vi "Thin Etalon Linewidth Sweep 2.0 user.vi"() -> ()   [LabVIEW 2013]
uses:
  Sweep Control.ctl
panel:
  out "time":dbl(graph)
  out "centers":T1(graph)
  out "Remote Find Center":bool
  out "sweep states":T2
  out "Loop Counter":i32
  in  "Stop Button":bool
  out "Done":bool
  in  "Find Center":bool
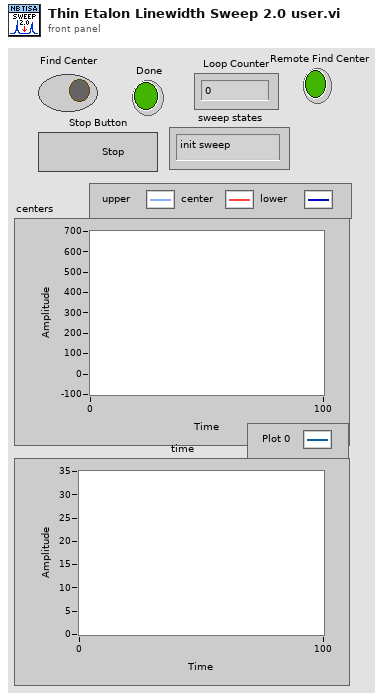
[diagram p1: front panel]
types:
  T1 = cluster{"Upper Limit":i32, "Center Position":i32, "Lower Limit":i32}
  T2 = typedef "Sweep Control.ctl" = enum16{"init sweep", "do sweep", "idle"}
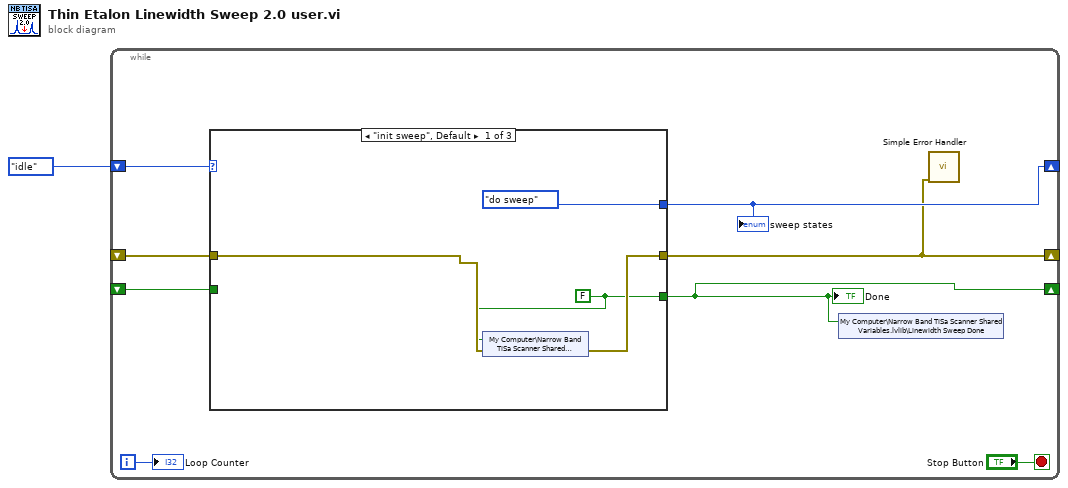
[diagram p0: block diagram]
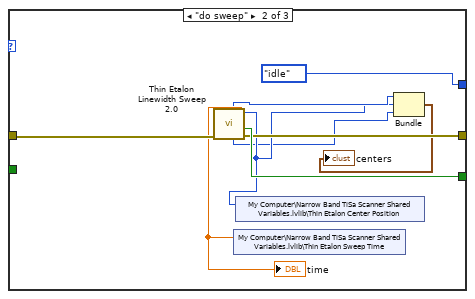
[diagram p2: hidden frame]
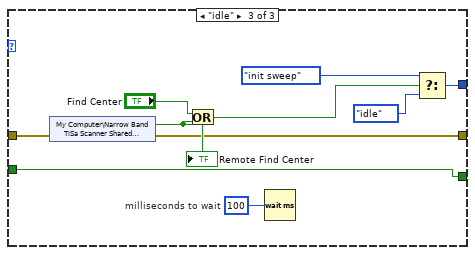
[diagram p3: hidden frame]
diagram:
  n1 = while {
    shift-right: [w5] -> _
    shift-left: Sweep_Control."idle" -> [w7]
    shift-right: [w2] -> _
    shift-left: _ -> [w6]
    shift-right: [w4] -> _
    shift-left: _ -> [w3]
    i -> [w8]
    stop <- "Stop Button" stop-if-true
    n2 = case shown="\"init sweep\", Default" w7 {
      tunnel: [w11 w20 w23] -> w2
      tunnel: w6 -> [w12 w21 w30]
      tunnel: [Sweep_Control."do sweep" Sweep_Control."idle" w26] -> w5
      tunnel: [w10 w22 w24] -> w4
      tunnel: w3 -> [_ _ w24]
      frame "init sweep", Default {
        w10 = FALSE
        n3 = shared-variable "My Computer\\Narrow Band TiSa Scanner Shared Variables.lvlib\\Find Center"(w10, error in=w12) -> (error out=w11:errorcluster)
      }
      frame "do sweep" {
        n4 = call "Thin Etalon Linewidth Sweep 2.0.vi"("Error In"=w21) -> ("Error Out"=w20:errorcluster, "Done"=w22:bool, "Time Elapsed"=w18:dbl, "Center Position"=w16:i32, "Lower Limit"=w15:i32, "Upper Limit"=w17:i32)  [unwired: 5 in]
        "time" <- w18
        n5 = shared-variable "My Computer\\Narrow Band TiSa Scanner Shared Variables.lvlib\\Thin Etalon Sweep Time"(w18) -> ()  [unwired: 1 in, 1 out]
        n6 = shared-variable "My Computer\\Narrow Band TiSa Scanner Shared Variables.lvlib\\Thin Etalon Center Position"(w16) -> ()  [unwired: 1 in, 1 out]
        n7 = Bundle("Upper Limit"=w17, "Center Position"=w16, "Lower Limit"=w15) -> (→"centers":T1)  [unwired: 1 in]
      }
      frame "idle" {
        w25 = u32 100  # milliseconds to wait
        n8 = shared-variable "My Computer\\Narrow Band TiSa Scanner Shared Variables.lvlib\\Find Center"(error in=w30) -> (w31:bool, error out=w23:errorcluster)
        "Remote Find Center" <- w31
        n9 = Or(x="Find Center", y=w31) -> (x .or. y?=w28:bool)
        n10 = Wait (ms)(milliseconds to wait=w25) -> ()  [unwired: 1 out]
        n11 = Select(t=Sweep_Control."init sweep", s=w28, f=Sweep_Control."idle") -> (s? t:f=w26:T2)
      }
    }
    "Done" <- w4
    "sweep states" <- w5
    n12 = shared-variable "My Computer\\Narrow Band TiSa Scanner Shared Variables.lvlib\\Linewidth Sweep Done"(w4) -> ()  [unwired: 1 in, 1 out]
    n13 = call <vilib>:"Simple Error Handler.vi"("error in (no error)"=w2) -> ()  [unwired: 4 in, 5 out]
    "Loop Counter" <- w8
  }
